vi "Script_32x32.vi"() -> ()   [LabVIEW 2011]
panel:
  out "Numeric 2":i32
  out "Numeric":i32
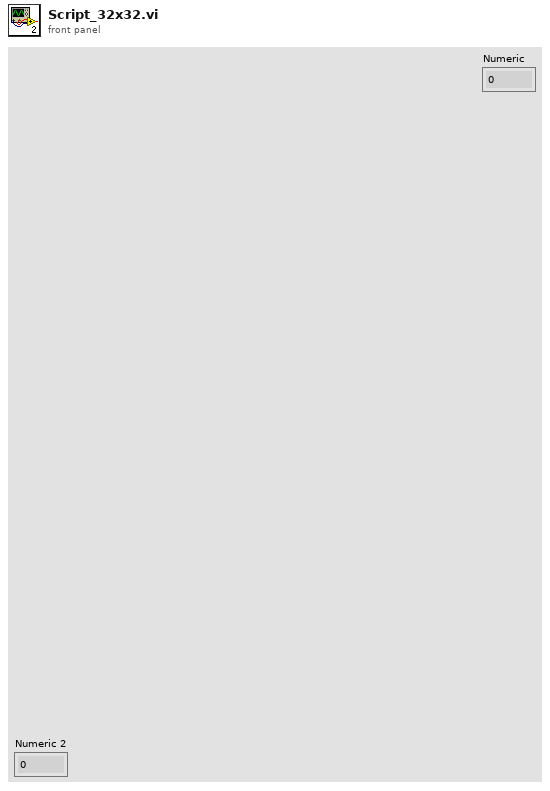
[diagram p1: front panel]
types:
  T1 = enum32{"Invalid", "Standard", "Closed", "Hidden", "Minimized", "Maximized"}
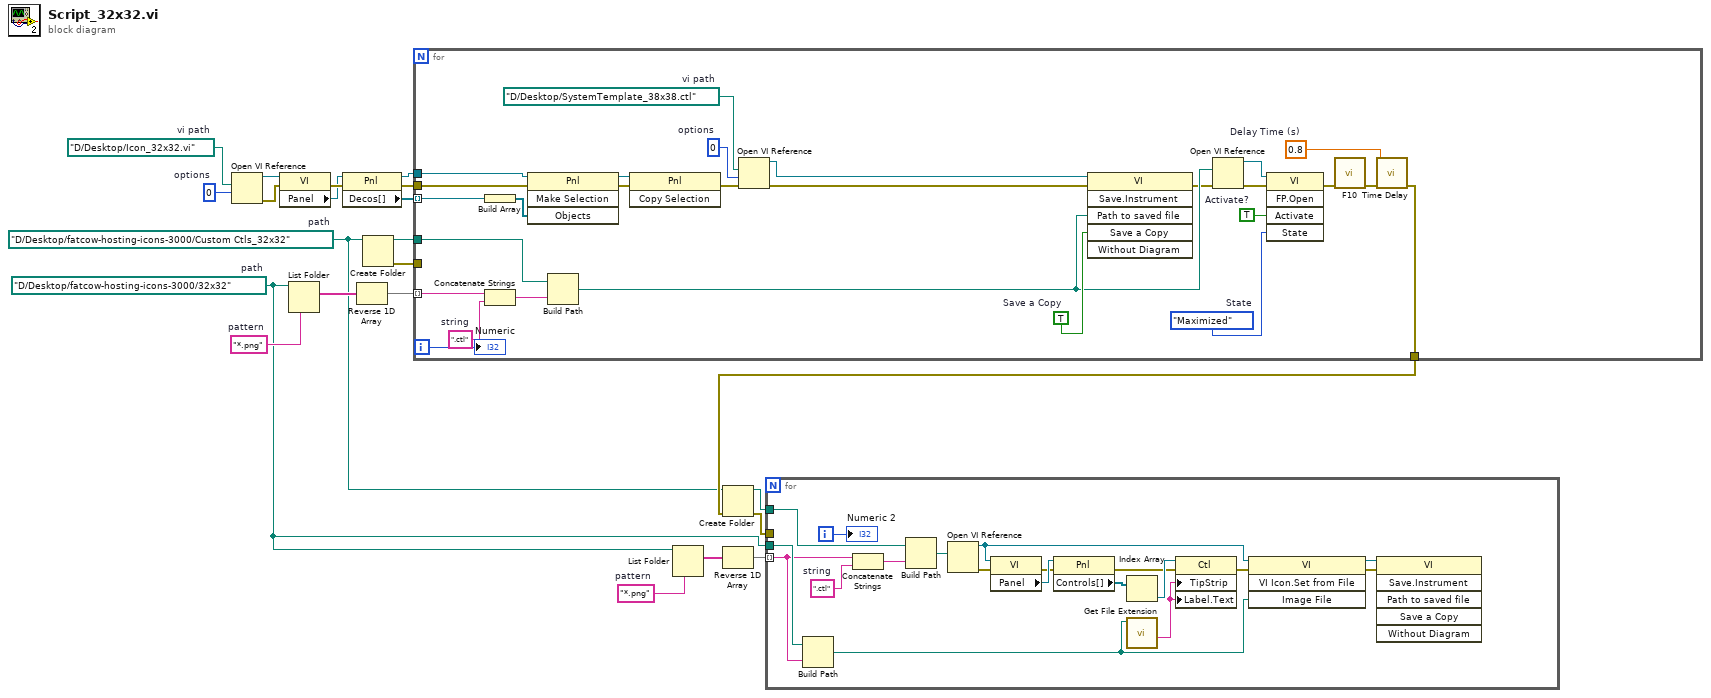
[diagram p0: block diagram]
diagram:
  w8 = "*.png"  # pattern
  w2 = path "D:/Desktop/fatcow-hosting-icons-3000/Custom Ctls_32x32"  # path
  w15 = "*.png"  # pattern
  w1 = path "D:/Desktop/fatcow-hosting-icons-3000/32x32"  # path
  w22 = path "D:/Desktop/Icon_32x32.vi"  # vi path
  w21 = 0  # options
  n1 = Open VI Reference(vi path=w22, options=w21) -> (vi reference=w13:refnum<vi>, error out=w12:errorcluster)  [unwired: 4 in]
  n2 = property class="VI"(reference=w13, error in=w12) -> (error out=w19:errorcluster, "Panel"=w16:refnum<vi>)  [unwired: 1 out]
  n3 = List Folder(path=w1, pattern=w15) -> (filenames=w14:string[])  [unwired: 2 in, 3 out]
  n4 = property class="Pnl"(reference=w16, error in=w19) -> (reference out=w18:refnum<vi>, error out=w17:errorcluster, "Decos[]"=w20:refnum<vi>[])
  n5 = Reverse 1D Array(array=w14) -> (reversed array=w9:string[])
  n6 = Create Folder(path (use dialog)=w2) -> (created path=w11:path, error out=w10:errorcluster)  [unwired: 2 in, 1 out]
  n7 = for {
    tunnel: w20 -> [w47] mode=indexing
    tunnel: w18 -> [w44]
    tunnel: w17 -> [w43]
    tunnel: w9 -> [w37] mode=indexing
    tunnel: w11 -> [w34]
    tunnel: w10 -> [_]
    tunnel: [w23] -> w3
    i -> [w24]
    w25 = 0.8  # Delay Time (s)
    w28 = T1."Maximized"  # State
    w30 = TRUE  # Activate?
    w36 = ".ctl"  # string
    w41 = TRUE  # Save a Copy
    w48 = path "D:/Desktop/SystemTemplate_38x38.ctl"  # vi path
    w49 = 0  # options
    n8 = Build Array(w47) -> (w38:refnum<vi>[])
    n9 = Concatenate Strings(w37, w36) -> (w35:string)
    n10 = invoke class="Pnl" method="Make Selection"(reference=w44, error in=w43, "Objects"=w38) -> (reference out=w46:refnum<vi>, error out=w42:errorcluster)  [unwired: 1 in, 2 out]
    n11 = Build Path(base path=w34, name or relative path=w35) -> (appended path=w33:path)
    n12 = invoke class="Pnl" method="Copy Selection"(reference=w46, error in=w42) -> (error out=w45:errorcluster)  [unwired: 1 in, 2 out]
    n13 = Open VI Reference(vi path=w48, options=w49, error in (no error)=w45) -> (vi reference=w40:refnum<vi>, error out=w39:errorcluster)  [unwired: 3 in]
    n14 = invoke class="VI" method="Save.Instrument"(reference=w40, error in=w39, "Path to saved file"=w33, "Save a Copy"=w41) -> (error out=w29:errorcluster)  [unwired: 2 in, 5 out]
    n15 = Open VI Reference(vi path=w33, error in (no error)=w29) -> (vi reference=w32:refnum<vi>, error out=w31:errorcluster)  [unwired: 4 in]
    n16 = invoke class="VI" method="FP.Open"(reference=w32, error in=w31, "Activate"=w30, "State"=w28) -> (error out=w27:errorcluster)  [unwired: 1 in, 4 out]
    n17 = call "F10.vi"("error in (no error)"=w27) -> ("error out"=w26:errorcluster)  [unwired: 10 in]
    n18 = call "Time Delay"("error in (no error)"=w26, "Delay Time (s)"=w25) -> ("error out"=w23:errorcluster)  [unwired: 9 in]
    "Numeric" <- w24
  }
  n19 = List Folder(path=w1, pattern=w8) -> (filenames=w7:string[])  [unwired: 2 in, 3 out]
  n20 = Create Folder(path (use dialog)=w2, error in=w3) -> (created path=w6:path, error out=w5:errorcluster)  [unwired: 1 in, 1 out]
  n21 = Reverse 1D Array(array=w7) -> (reversed array=w4:string[])
  n22 = for {
    tunnel: w4 -> [w63] mode=indexing
    tunnel: w6 -> [w66]
    tunnel: w5 -> [_]
    tunnel: w1 -> [w64]
    i -> [w55]
    w68 = ".ctl"  # string
    n23 = Build Path(base path=w64, name or relative path=w63) -> (appended path=w57:path)
    n24 = Concatenate Strings(w63, w68) -> (w67:string)
    n25 = Build Path(base path=w66, name or relative path=w67) -> (appended path=w65:path)
    n26 = Open VI Reference(vi path=w65) -> (vi reference=w61:refnum<vi>, error out=w51:errorcluster)  [unwired: 5 in]
    n27 = property class="VI"(reference=w61, error in=w51) -> (error out=w54:errorcluster, "Panel"=w60:refnum<vi>)  [unwired: 1 out]
    n28 = property class="Pnl"(reference=w60, error in=w54) -> (error out=w53:errorcluster, "Controls[]"=w59:refnum<vi>[])  [unwired: 1 out]
    n29 = Index Array(array=w59) -> (element=w58:refnum<vi>)  [unwired: 1 in]
    n30 = call <vilib>:"Get File Extension.vi"("file"=w57) -> ("filename without extension"=w56:string)  [unwired: 7 in, 3 out]
    n31 = property class="Ctl"(reference=w58, error in=w53, "TipStrip"=w56, "Label.Text"=w56) -> (error out=w52:errorcluster)  [unwired: 1 out]
    n32 = invoke class="VI" method="VI Icon.Set from File"(reference=w61, error in=w52, "Image File"=w57) -> (reference out=w62:refnum<vi>, error out=w50:errorcluster)  [unwired: 1 in, 2 out]
    n33 = invoke class="VI" method="Save.Instrument"(reference=w62, error in=w50) -> ()  [unwired: 4 in, 6 out]
    "Numeric 2" <- w55
  }
